vi "bubble.vi"(3 "Direction":bool, 4 "in":dbl[](array[numeric])) -> (0 "counter":i32, 1 "out":dbl[](array[numeric]))   [LabVIEW 2024]
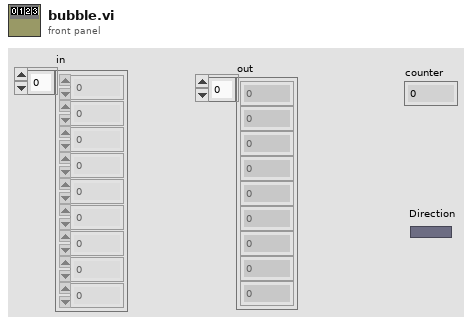
[diagram p1: front panel]
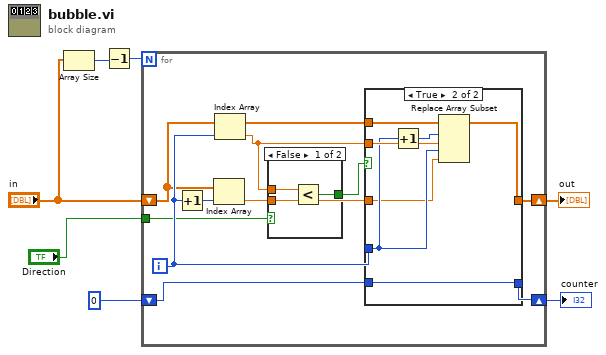
[diagram p0: block diagram]
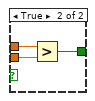
[diagram p2: hidden frame]
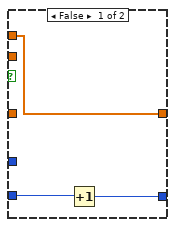
[diagram p3: hidden frame]
diagram:
  n1 = Array Size(array="in") -> (size(s)=w6:i32)
  n2 = Decrement(x=w6) -> (x-1=w5:i32)
  n3 = for {
    N: w5 -> [_]
    shift-right: [w14] -> w4
    shift-left: "in" -> [w15]
    shift-right: [w12] -> w2
    shift-left: 0 -> [w13]
    tunnel: "Direction" -> [w11]
    i -> [w16]
    n4 = Increment(x=w16) -> (x+1=w17:i32)
    n5 = Index Array(array=w15, index=w17) -> (element=w10:dbl)
    n6 = Index Array(array=w15, index=w16) -> (element=w9:dbl)
    n7 = case shown="False" w11 {
      tunnel: w10 -> [w18 w23]
      tunnel: w9 -> [w19 w22]
      tunnel: [w20 w21] -> w8
      frame False {
        n8 = Less?(x=w19, y=w18) -> (x < y?=w20:bool)
      }
      frame True {
        n9 = Greater?(x=w22, y=w23) -> (0:w21:bool)
      }
    }
    n10 = case shown="True" w8 {
      tunnel: w16 -> [_ w31]
      tunnel: w15 -> [w26 w33]
      tunnel: w9 -> [_ w32]
      tunnel: [w26 w29] -> w14
      tunnel: w13 -> [w25 w28]
      tunnel: [w24 w28] -> w12
      tunnel: w10 -> [_ w27]
      frame False {
        n11 = Increment(x=w25) -> (x+1=w24:i32)
      }
      frame True {
        n12 = Increment(x=w31) -> (x+1=w30:i32)
        n13 = Replace Array Subset(array=w33, new element #1=w32, index #1=w30, new element #2=w27, index #2=w31) -> (w29:dbl[])
      }
    }
  }
  "out" <- w4
  "counter" <- w2
